vi "Myrio_2.vi"   [LabVIEW 2012]
uses:
  SubVIs/LVPresent_Globals.vi
panel:
  # "Get to know the board"
  # "The myRIO has four onboard LEDs, which you can control."
  # "There are two audio ports on the side."
  # "It has two connectors for an external breakout board."
  # "There is a set of connectors  for indivual wires."
  # "There are also accelerometers inside of the myRIO"
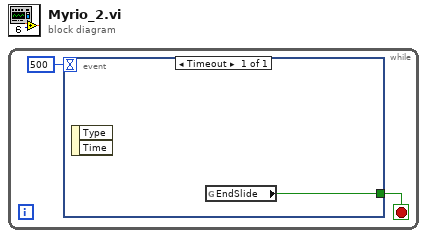
[diagram p0: block diagram]
diagram:
  n1 = while {
    stop <- w2 stop-if-true
    n2 = event shown="[0] Timeout" {
      selector: _ -> [_]
      dyn-events: _ -> [_]
      timeout: 500 -> [_]
      tunnel: [w3] -> w2
      event Timeout {
        n3 = event-data() -> ()  [unwired: 1 in, 2 out]
        n4 = global read "LVPresent_Globals.vi" "EndSlide"() -> (w3:bool)
      }
    }
  }
